vi "Configure Modulation Waveform (Noise).vi"(6 "Noise Type (0: Uniform)":u16(ring) items=["Uniform", "Gaussian"], 7 "Modulation Path (1)":u16(ring)=1 items=["1"=1, "2"=2], 8 "error in (no error)":errorcluster, 9 "Internal Source (1)":u16(ring)=1 items=["1"=1, "2"=2], 10 "Modulation Type (0: Amplitude Modulation)":u16(ring) items=["Amplitude Modulation", "Frequency Modulation", "Phase Modulation", "Low Frequency Output"], 11 "VISA resource name":refnum<visa-resource-name>) -> (0 "error out":errorcluster, 3 "VISA resource name out":refnum<visa-resource-name>)   [LabVIEW 2018, in "Agilent PSG MXG Series.lvlib"]
doc: "Configures the noise type for the noise waveform.\n\n<B>Notes:</B>\n(1) This VI is <B>NOT</B> valid in E8247C, N5161A, N5162A, N5181A, N5182A, N5183A.\n\n(2) For E8257D, E8267D, this VI is valid only when the instrument installs <B>Option UNT</B> (AM, FM, phase modulation, and LF output).\n\n(3) For N5171B, N5172B, N5181B, N5182B, N5173B, N5183B, this VI is valid only when the instrument installs <B>Option UNT</B> and <B>Option 303</B> (AM, FM, phase modulation, and LF output)."
uses:
  Agilent PSG MXG Series.lvlib
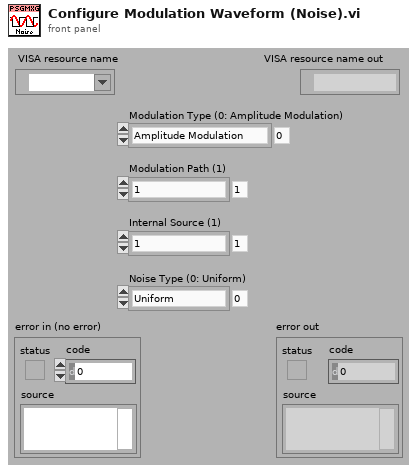
[diagram p1: front panel]
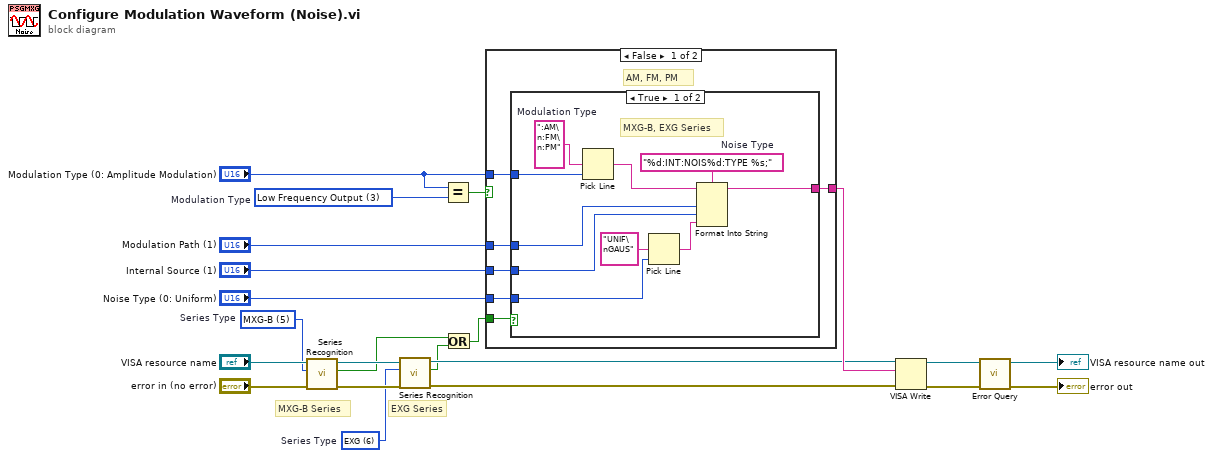
[diagram p0: block diagram]
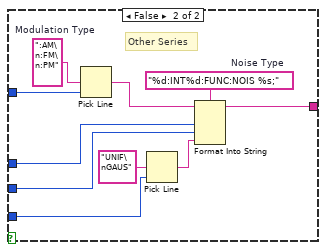
[diagram p2: hidden frame]
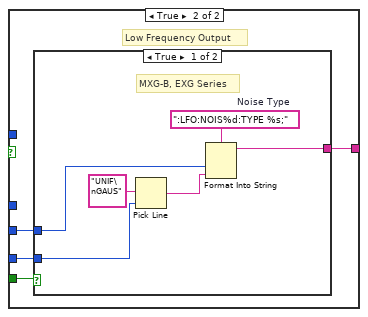
[diagram p3: hidden frame]
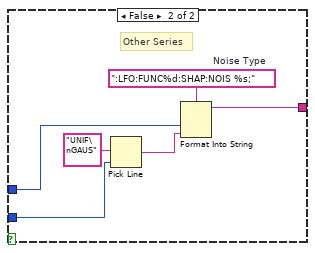
[diagram p4: hidden frame]
diagram:
  w1 = u16 3 items=["Amplitude Modulation", "Frequency Modulation", "Phase Modulation", "Low Frequency Output"]  # Modulation Type
  w7 = u16 6 items=["MXG-A", "PSG", "PSG-A", "PSG-C", "PSG-D", "MXG-B", "EXG"]  # Series Type
  w10 = u16 5 items=["MXG-A", "PSG", "PSG-A", "PSG-C", "PSG-D", "MXG-B", "EXG"]  # Series Type
  # "EXG Series"
  # "MXG-B Series"
  n1 = call "Series Recognition.vi"("error in (no error)"="error in (no error)", "Series Type (0: MXG)"=w10, "VISA resource name"="VISA resource name") -> ("error out"=w8:errorcluster, "Is Series Correct"=w6:bool, "VISA resource name out"=w9:refnum<visa-resource-name>)  [unwired: 6 out]
  n2 = call "Series Recognition.vi"("error in (no error)"=w8, "Series Type (0: MXG)"=w7, "VISA resource name"=w9) -> ("error out"=w4:errorcluster, "Is Series Correct"=w3:bool, "VISA resource name out"=w5:refnum<visa-resource-name>)  [unwired: 6 out]
  n3 = Equal?(x="Modulation Type (0: Amplitude Modulation)", y=w1) -> (x = y?=w22:bool)
  n4 = Or(x=w6, y=w3) -> (x .or. y?=w2:bool)
  n5 = case shown="False" w22 {
    tunnel: "Modulation Type (0: Amplitude Modulation)" -> [w28 _]
    tunnel: "Modulation Path (1)" -> [w27 _]
    tunnel: "Internal Source (1)" -> [w26 w52]
    tunnel: "Noise Type (0: Uniform)" -> [w25 w51]
    tunnel: [w24 w50] -> w17
    tunnel: w2 -> [w23 w49]
    frame False {
      # "AM, FM, PM"
      n6 = case shown="True" w23 {
        tunnel: w28 -> [w35 w45]
        tunnel: w27 -> [w34 w44]
        tunnel: w26 -> [w33 w43]
        tunnel: w25 -> [w31 w41]
        tunnel: [w29 w39] -> w24
        frame True {
          w37 = "%d:INT:NOIS%d:TYPE %s;"  # Noise Type
          w38 = ":AM\n:FM\n:PM"  # Modulation Type
          # "MXG-B, EXG Series"
          n7 = Pick Line(multi-line string=w38, line index=w35) -> (output string=w36:string)  [unwired: 1 out]
          n8 = Pick Line(multi-line string="UNIF\nGAUS", line index=w31) -> (output string=w30:string)  [unwired: 1 out]
          n9 = Format Into String(format string=w37, initial string=w36, w34, w33, w30) -> (resulting string=w29:string)  [unwired: 1 in, 1 out]
        }
        frame False {
          w47 = "%d:INT%d:FUNC:NOIS %s;"  # Noise Type
          w48 = ":AM\n:FM\n:PM"  # Modulation Type
          # "Other Series"
          n10 = Pick Line(multi-line string=w48, line index=w45) -> (output string=w46:string)  [unwired: 1 out]
          n11 = Pick Line(multi-line string="UNIF\nGAUS", line index=w41) -> (output string=w40:string)  [unwired: 1 out]
          n12 = Format Into String(format string=w47, initial string=w46, w44, w43, w40) -> (resulting string=w39:string)  [unwired: 1 in, 1 out]
        }
      }
    }
    frame True {
      # "Low Frequency Output"
      n13 = case shown="True" w49 {
        tunnel: w52 -> [w57 w63]
        tunnel: w51 -> [w55 w61]
        tunnel: [w53 w59] -> w50
        frame True {
          w58 = ":LFO:NOIS%d:TYPE %s;"  # Noise Type
          # "MXG-B, EXG Series"
          n14 = Pick Line(multi-line string="UNIF\nGAUS", line index=w55) -> (output string=w54:string)  [unwired: 1 out]
          n15 = Format Into String(format string=w58, w57, w54) -> (resulting string=w53:string)  [unwired: 2 in, 1 out]
        }
        frame False {
          w64 = ":LFO:FUNC%d:SHAP:NOIS %s;"  # Noise Type
          # "Other Series"
          n16 = Pick Line(multi-line string="UNIF\nGAUS", line index=w61) -> (output string=w60:string)  [unwired: 1 out]
          n17 = Format Into String(format string=w64, w63, w60) -> (resulting string=w59:string)  [unwired: 2 in, 1 out]
        }
      }
    }
  }
  n18 = VISA Write(VISA resource name=w5, write buffer=w17, error in (no error)=w4) -> (VISA resource name out=w16:refnum<visa-resource-name>, error out=w15:errorcluster)  [unwired: 1 out]
  n19 = call "Error Query.vi"("error in (no error)"=w15, "VISA resource name"=w16) -> ("error out"=→"error out":errorcluster, "VISA resource name out"=→"VISA resource name out":refnum<visa-resource-name>)  [unwired: 8 out]
